vi "PressureReadingsChanged.vi"(8 "error in (no error)":errorcluster, 11 "senseHatSensors in":refnum<class "RPI.SenseHat.Sensors.lvclass">) -> (0 "error out":errorcluster, 3 "senseHatSensors out":refnum<class "RPI.SenseHat.Sensors.lvclass">)   [LabVIEW 2020, in "RPI.SenseHat.Sensors.lvlib" / "RPI.SenseHat.Sensors.lvclass"]
uses:
  RPI.SenseHat.Sensors.lvclass
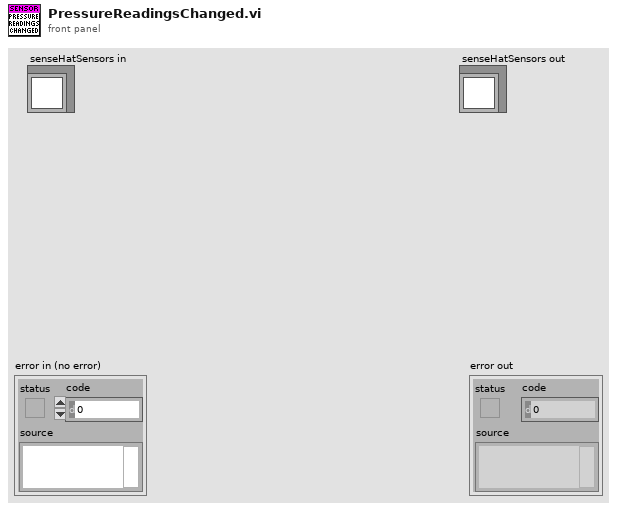
[diagram p1: front panel]
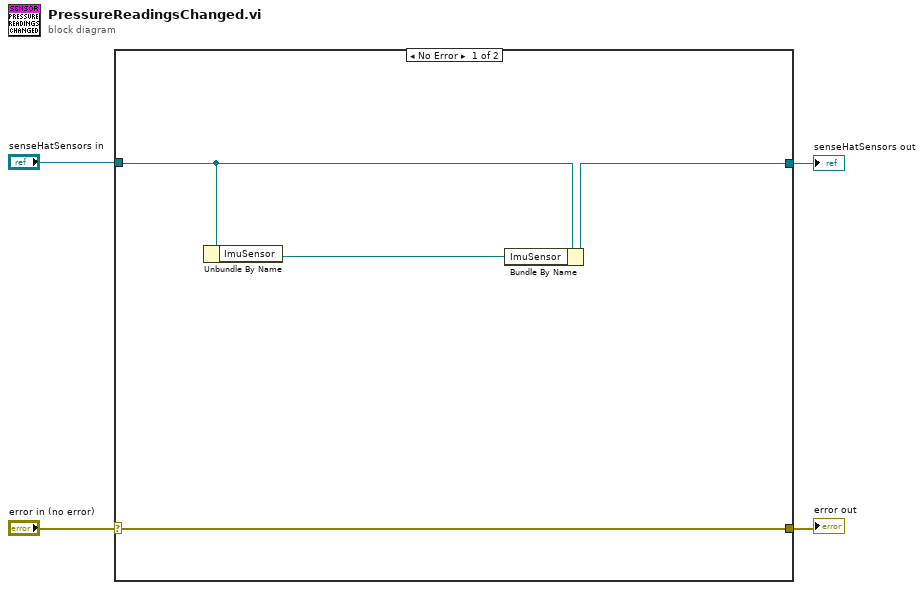
[diagram p0: block diagram]
diagram:
  n1 = case shown="No Error" "error in (no error)" {
    selector: "error in (no error)" -> [w7 w10]
    tunnel: [w7 w10] -> w3
    tunnel: [w5 w9] -> w1
    tunnel: "senseHatSensors in" -> [w6 w9]
    frame No Error {
      n2 = Unbundle By Name(w6) -> ("ImuSensor"=w8:refnum<class "imuSensor.lvclass">)
      n3 = Bundle By Name(cluster=w6, "ImuSensor"=w8) -> (w5:refnum<class "RPI.SenseHat.Sensors.lvclass">)
    }
    frame Error {
    }
  }
  "error out" <- w3
  "senseHatSensors out" <- w1
